vi "UV_LED switch.vi"(6 "ForceOff":bool, 7 "On/Off (F:off)":bool, 8 "error in":errorcluster, 10 "CHN":T1 items=["All", "CH1", "CH2", "CH3", "CH4"], 11 "VISA resource":refnum<visa-resource-name>) -> (0 "error out":errorcluster, 2 "CH_change":u8, 3 "VISA resource out":refnum<visa-resource-name>, 5 "Err?":bool)   [LabVIEW 8.6]
uses:
  TypeDef/UVLed_func.ctl
  TypeDef/UVLed_channel.ctl
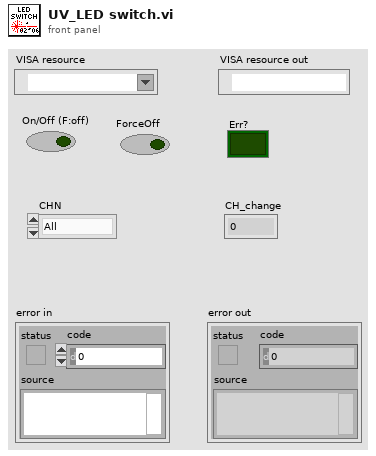
[diagram p1: front panel]
types:
  T1 = typedef "UVLed_channel.ctl" = u16
  T2 = typedef "UVLed_func.ctl" = u16
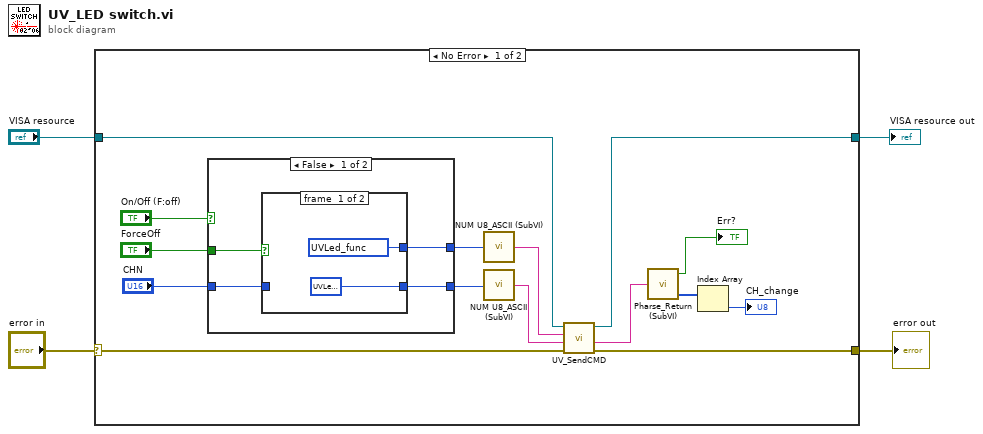
[diagram p0: block diagram]
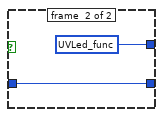
[diagram p2: hidden frame]
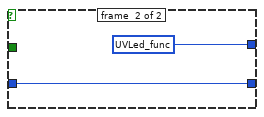
[diagram p3: hidden frame]
diagram:
  n1 = case shown="No Error" "error in" {
    selector: "error in" -> [w16 w31]
    tunnel: [w14 w31] -> w3
    tunnel: "VISA resource" -> [w17 w30]
    tunnel: [w12 w30] -> w1
    frame #0 {
      n2 = case shown="False" "On/Off (F:off)" {
        tunnel: [w23 w29] -> w19
        tunnel: "CHN" -> [w20 w28]
        tunnel: [w21 w28] -> w10
        tunnel: "ForceOff" -> [w22 _]
        frame #0 {
          n3 = case shown="False" w22 {
            tunnel: [w25 w27] -> w23
            tunnel: [w24 w26] -> w21
            tunnel: w20 -> [_ w26]
            frame #0 {
              w24 = T1 ? items=["All", "CH1", "CH2", "CH3", "CH4"] ("CHN")
              w25 = T2 ? items=["GetAllStatus", "LightOn", "LightOff", "AllForceOff", "GetMenuChnPara", "SetMenuChnPara", "GetAutoChnPara", "SetAutoChnPara", "GetMenuTemplate", "SetMenuTemplate", "GetAutoTemplate", "SetAutoTemplate", "GetTemplatePara", "SetTemplatePara", "GetMode", "SetMode", "ChkErr"] ("Function")
            }
            frame #1 {
              w27 = T2 ? items=["GetAllStatus", "LightOn", "LightOff", "AllForceOff", "GetMenuChnPara", "SetMenuChnPara", "GetAutoChnPara", "SetAutoChnPara", "GetMenuTemplate", "SetMenuTemplate", "GetAutoTemplate", "SetAutoTemplate", "GetTemplatePara", "SetTemplatePara", "GetMode", "SetMode", "ChkErr"] ("Function")
            }
          }
        }
        frame #1 {
          w29 = T2 ? items=["GetAllStatus", "LightOn", "LightOff", "AllForceOff", "GetMenuChnPara", "SetMenuChnPara", "GetAutoChnPara", "SetAutoChnPara", "GetMenuTemplate", "SetMenuTemplate", "GetAutoTemplate", "SetAutoTemplate", "GetTemplatePara", "SetTemplatePara", "GetMode", "SetMode", "ChkErr"] ("Function")
        }
      }
      n4 = call "NUM U8_ASCII (SubVI).vi"("Numeric"=w19) -> ("String out"=w18:string)
      n5 = call "NUM U8_ASCII (SubVI).vi"("Numeric"=w10) -> ("String out"=w15:string)
      n6 = call "UV_SendCMD.vi"("error in"=w16, "value"=w15, "function"=w18, "VISA resource name"=w17) -> ("error out"=w14:errorcluster, "response"=w13:string, "VISA resource name out"=w12:refnum<visa-resource-name>)  [unwired: 5 in]
      n7 = call "Pharse_Return (SubVI).vi"("buffer in"=w13) -> ("byte array"=w6:u8[], "Err?"=→"Err?":bool)  [unwired: 2 in, 1 out]
      n8 = Index Array(array=w6) -> (element=→"CH_change":u8)  [unwired: 1 in]
    }
    frame #1 {
    }
  }
  "error out" <- w3
  "VISA resource out" <- w1
